vi "Read user Messages.vi"(8 "error in (no error)":errorcluster) -> (0 "error out":errorcluster, 3 "ATM Messages":T1)   [LabVIEW 2018, in "Controller.lvlib"]
doc: "Reads atm messages from txt file."
uses:
  Controller.lvlib
  Module Data.ctl
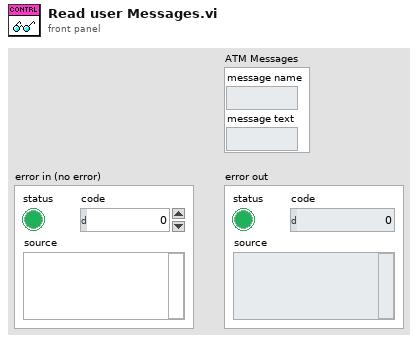
[diagram p1: front panel]
types:
  T1 = typedef "Controller.lvlib/Module Data.ctl" = cluster{"message name":string, "message text":string}
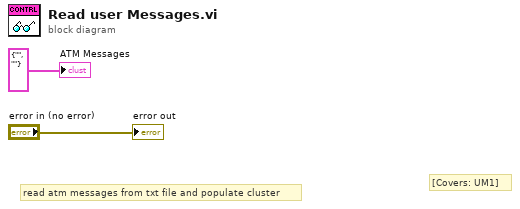
[diagram p0: block diagram]
diagram:
  # "[Covers: UM1]"
  # "read atm messages from txt file and populate cluster"
  "error out" <- "error in (no error)"
  "ATM Messages" <- T1 {"message name"="", "message text"=""} ("ATM Messages")
